vi "Convert to SSE.vi"(5 "Check Query Parameters for lastEventId? (true)":bool=TRUE, 7 "Add Wildcard CORS Header? (true)":bool=TRUE, 8 "Error In":errorcluster, 11 "LabVIEW Web Service Request In":refnum<class "Web Request.lvclass">) -> (0 "Error Out":errorcluster, 1 "Last Event ID found?":bool, 2 "Last Event ID":string, 3 "LabVIEW Web Service Request Out":refnum<class "Web Request.lvclass">)   [LabVIEW 2014, in "i3-sse-server.lvlib"]
uses:
  i3-sse-server.lvlib
  <vilib>/wsapi/Web Request.lvclass
  <vilib>/Utility/error.llb/Error Cluster From Error Code.vi
  <vilib>/ErrorRing/Error Ring.xnode
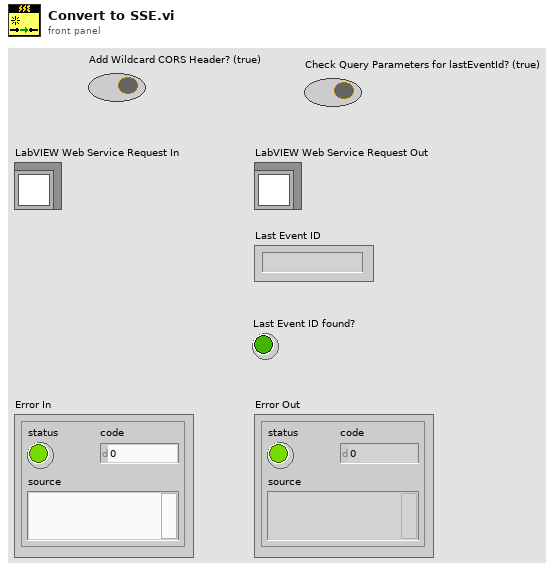
[diagram p1: front panel]
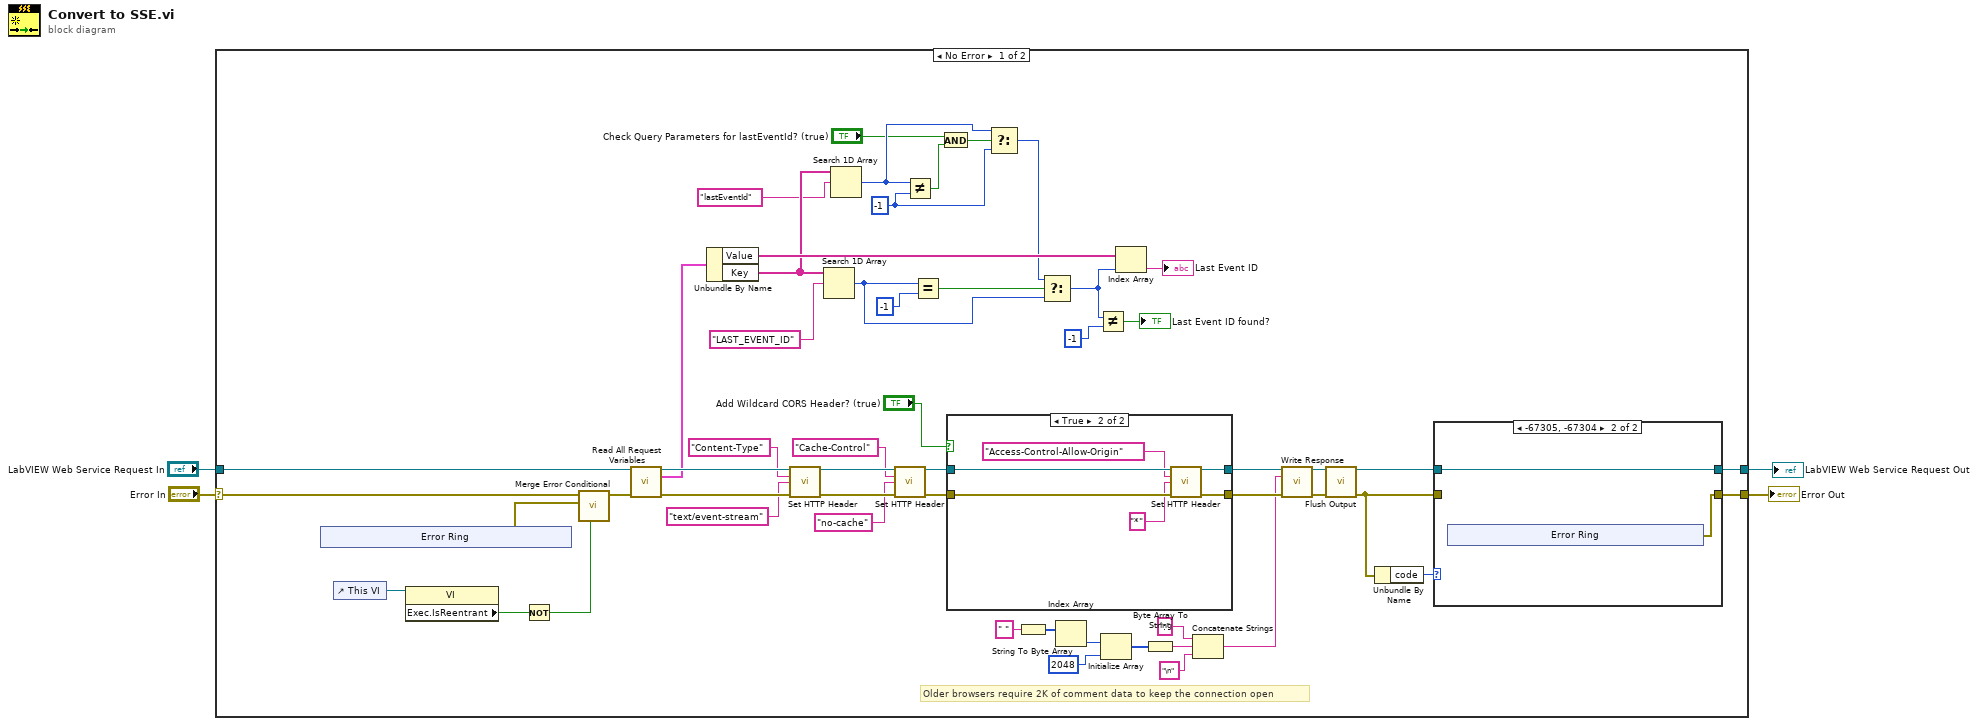
[diagram p0: block diagram]
diagram:
  n1 = case shown="No Error" "Error In" {
    selector: "Error In" -> [w8 w82]
    tunnel: "LabVIEW Web Service Request In" -> [w38 w81]
    tunnel: [w28 w82] -> w2
    tunnel: [w26 w81] -> w1
    frame No Error {
      w45 = -1 ("y")
      # "Older browsers require 2K of comment data to keep the connection open"
      n2 = xnode "Error Ring"() -> ("error out"=w7:errorcluster)
      n3 = control-ref of="This VI"() -> (w54:refnum<vi>)
      n4 = property class="VI"(reference=w54) -> ("Exec.IsReentrant"=w6:bool)  [unwired: 1 in, 2 out]
      n5 = Not(x=w6) -> (.not. x?=w5:bool)
      n6 = call "Merge Error Conditional.vi"("Merge Error? (true)"=w5, "Error To Merge"=w7, "Original Error Wire"=w8) -> ("Error Out"=w9:errorcluster)  [unwired: 8 in]
      n7 = call <vilib>:"Read All Request Variables.vi"("LabVIEW Web Service Request"=w38, "error in (no error)"=w9) -> ("LabVIEW Web Service Request out"=w58:refnum<class "Web Request.lvclass">, "request variables"=w53:cluster{"Key":string[], "Value":string[]}, "error out"=w37:errorcluster)  [unwired: 11 in]
      n8 = Unbundle By Name(w53) -> ("Value"=w57:string[], "Key"=w55:string[])
      n9 = call <vilib>:"Set HTTP Header.vi"("LabVIEW Web Service Request"=w58, "header"="Content-Type", "header value"="text/event-stream", "error in (no error)"=w37) -> ("LabVIEW Web Service Request out"=w34:refnum<class "Web Request.lvclass">, "error out"=w33:errorcluster)  [unwired: 10 in]
      n10 = Search 1D Array(1D array=w55, element="LAST_EVENT_ID") -> (index of element=w49:i32)  [unwired: 1 in]
      n11 = Search 1D Array(1D array=w55, element="lastEventId") -> (index of element=w56:i32)  [unwired: 1 in]
      n12 = call <vilib>:"Set HTTP Header.vi"("LabVIEW Web Service Request"=w34, "header"="Cache-Control", "header value"="no-cache", "error in (no error)"=w33) -> ("LabVIEW Web Service Request out"=w24:refnum<class "Web Request.lvclass">, "error out"=w23:errorcluster)  [unwired: 10 in]
      n13 = Not Equal?(x=w56, y=w45) -> (x != y?=w47:bool)
      n14 = Equal?(x=w49, y=-1) -> (x = y?=w50:bool)
      n15 = And(x="Check Query Parameters for lastEventId? (true)", y=w47) -> (x .and. y?=w46:bool)
      n16 = case shown="True" "Add Wildcard CORS Header? (true)" {
        tunnel: [w60 w66] -> w20
        tunnel: w24 -> [w60 w64]
        tunnel: w23 -> [w59 w63]
        tunnel: [w59 w65] -> w19
        frame False {
        }
        frame True {
          n17 = call <vilib>:"Set HTTP Header.vi"("LabVIEW Web Service Request"=w64, "header"="Access-Control-Allow-Origin", "header value"="*" ("header"), "error in (no error)"=w63) -> ("LabVIEW Web Service Request out"=w66:refnum<class "Web Request.lvclass">, "error out"=w65:errorcluster)  [unwired: 10 in]
        }
      }
      n18 = Select(t=w56, s=w46, f=w45) -> (s? t:f=w44:i32)
      n19 = String To Byte Array(string=" ") -> (unsigned byte array=w17:u8[])
      n20 = Select(t=w44, s=w50, f=w49) -> (s? t:f=w41:i32)
      n21 = Index Array(array=w17) -> (element=w16:u8)  [unwired: 1 in]
      n22 = Not Equal?(x=w41, y=-1) -> (x != y?=→"Last Event ID found?":bool)
      n23 = Initialize Array(w16, 2048 ("dimension size")) -> (w14:u8[])
      n24 = Index Array(array=w57, index=w41) -> (element=→"Last Event ID":string)
      n25 = Byte Array To String(unsigned byte array=w14) -> (string=w13:string)
      n26 = Concatenate Strings(":" ("string"), w13, "\n" ("string")) -> (w10:string)
      n27 = call <vilib>:"Write Response.vi"("LabVIEW Web Service Request"=w20, "response string"=w10, "error in (no error)"=w19) -> ("LabVIEW Web Service Request out"=w21:refnum<class "Web Request.lvclass">, "error out"=w22:errorcluster)  [unwired: 11 in]
      n28 = call <vilib>:"Flush Output.vi"("LabVIEW Web Service Request"=w21, "error in (no error)"=w22) -> ("LabVIEW Web Service Request out"=w27:refnum<class "Web Request.lvclass">, "error out"=w29:errorcluster)  [unwired: 12 in]
      n29 = Unbundle By Name(w29) -> ("code"=w30:i32)
      n30 = case shown="-67305, -67304" w30 {
        tunnel: w29 -> [w68 _]
        tunnel: [w68 w70] -> w28
        tunnel: w27 -> [w67 w69]
        tunnel: [w67 w69] -> w26
        frame Default {
        }
        frame -67305, -67304 {
          n31 = xnode "Error Ring"() -> ("error out"=w70:errorcluster)
        }
      }
    }
    frame Error {
    }
  }
  "Error Out" <- w2
  "LabVIEW Web Service Request Out" <- w1
